vi "ProgramGlobalReg.vi"(7 "Global Reg":u32[](array[numeric])=[68228136, 235670073, 4294967264, 4294967295, 4294967295, 511] format="%x", 8 "error in (no error)":errorcluster, 9 "ChipID":u32=65535 format="%x", 10 "LayerID":u32=65535 format="%x", 11 "connection ID":refnum<k5>) -> (0 "error out":errorcluster, 1 "OK?":bool, 2 "GlobalReg programmed":u32[](array[numeric]) format="%08x", 3 "connection ID out":refnum<k5>, 4 "Program done":string[](array[string]))   [LabVIEW 2015, in "VIPM2.lvlib"]
doc: "Fa la comprovació en tots els casos (emmascarant els ChipIDs)."
uses:
  VIPM2.lvlib
panel:
  out "Ready to receive data":string
  # "Program Global Register"
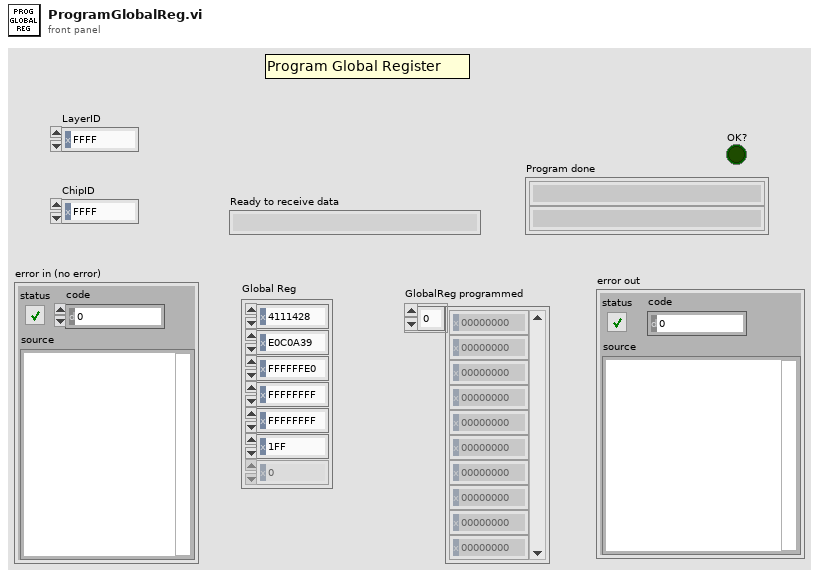
[diagram p1: front panel]
types:
  T1 = enum16{"Standard", "Buffered", "CRLF", "Immediate"}
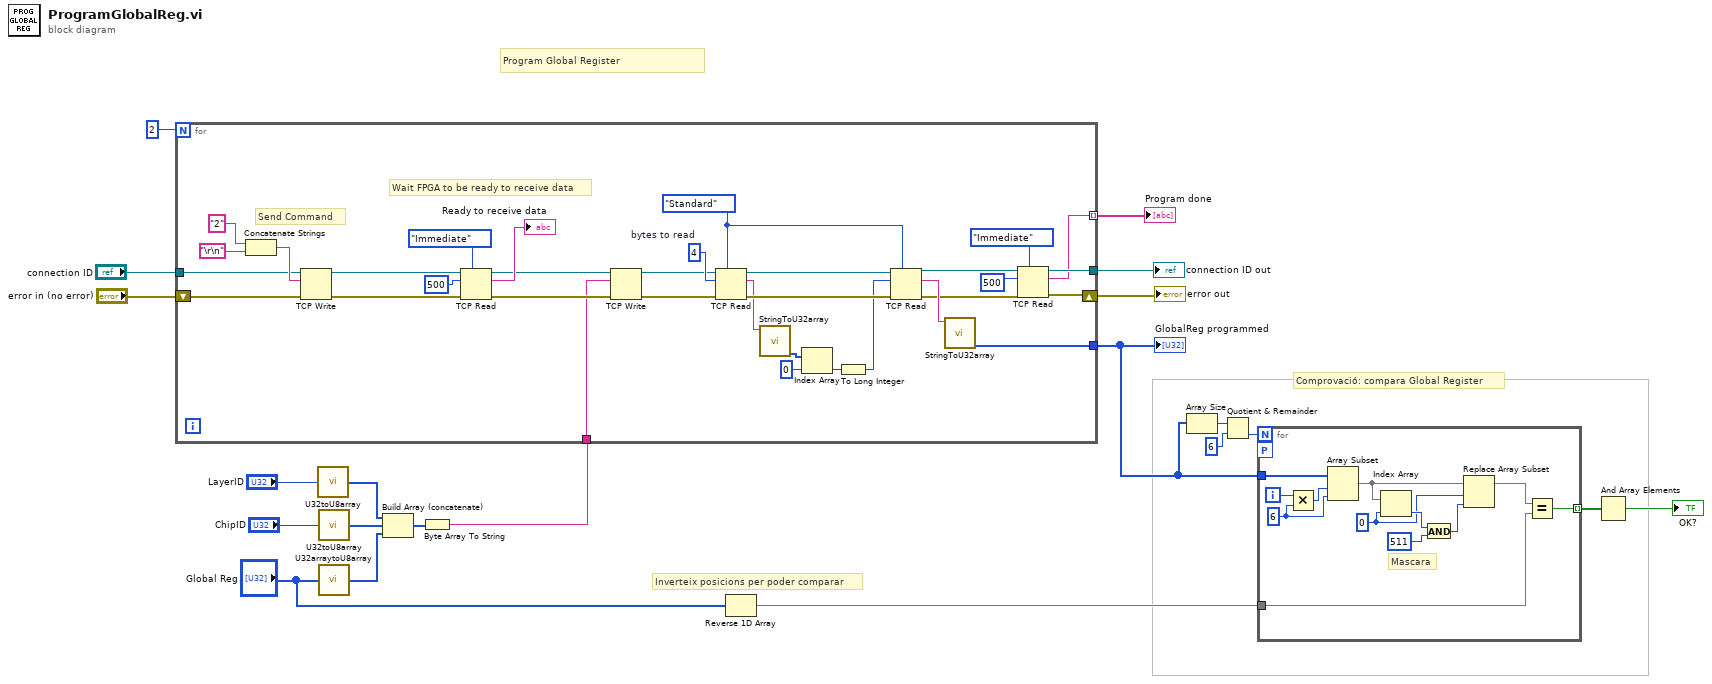
[diagram p0: block diagram]
diagram:
  # "Comprovació: compara Global Register"
  # "Inverteix posicions per poder comparar"
  # "Program Global Register"
  n1 = call "U32toU8array.vi"("x"="LayerID") -> ("ArrayU8"=w17:u8[])
  n2 = call "U32toU8array.vi"("x"="ChipID") -> ("ArrayU8"=w16:u8[])
  n3 = call "U32arraytoU8array.vi"("ArrayU32"="Global Reg") -> ("ArrayU8"=w15:u8[])
  n4 = Build Array (concatenate)(w17, w16, w15) -> (w18:u8[])
  n5 = Byte Array To String(unsigned byte array=w18) -> (string=w14:string)
  n6 = for {
    N: 2 -> [_]
    tunnel: "connection ID" -> [w51]
    tunnel: [w43] -> w20
    tunnel: [w42] -> w11 mode=indexing
    tunnel: w14 -> [w39]
    shift-right: [w25] -> w12
    shift-left: "error in (no error)" -> [w26]
    tunnel: [w24] -> w9
    w34 = 4  # bytes to read
    w35 = T1."Standard" ("mode (standard)")
    # "Wait FPGA to be ready to receive data"
    # "Send Command"
    n7 = Concatenate Strings("2" ("string"), "\r\n") -> (w52:string)
    n8 = TCP Write(connection ID=w51, data in=w52, error in (no error)=w26) -> (connection ID out=w47:refnum<k5>, error out=w46:errorcluster)  [unwired: 1 in, 1 out]
    n9 = TCP Read(connection ID=w47, bytes to read=500, error in (no error)=w46, 7:T1."Immediate" ("mode (standard)")) -> (connection ID out=w41:refnum<k5>, data out=→"Ready to receive data":string, error out=w40:errorcluster)  [unwired: 1 in]
    n10 = TCP Write(connection ID=w41, data in=w39, error in (no error)=w40) -> (connection ID out=w32:refnum<k5>, error out=w33:errorcluster)  [unwired: 1 in, 1 out]
    n11 = TCP Read(connection ID=w32, bytes to read=w34, error in (no error)=w33, 7:w35) -> (connection ID out=w38:refnum<k5>, data out=w31:string, error out=w37:errorcluster)  [unwired: 1 in]
    n12 = call "StringToU32array.vi"("String"=w31) -> ("U32array"=w30:u32[])  [unwired: 2 out]
    n13 = Index Array(array=w30, index=0) -> (element=w23:u32)
    n14 = To Long Integer(number=w23) -> (32bit integer=w22:i32)
    n15 = TCP Read(connection ID=w38, bytes to read=w22, error in (no error)=w37, 7:w35) -> (connection ID out=w28:refnum<k5>, data out=w29:string, error out=w27:errorcluster)  [unwired: 1 in]
    n16 = call "StringToU32array.vi"("String"=w29) -> ("U32array"=w24:u32[])  [unwired: 2 out]
    n17 = TCP Read(connection ID=w28, bytes to read=500, error in (no error)=w27, 7:T1."Immediate" ("mode (standard)")) -> (connection ID out=w43:refnum<k5>, data out=w42:string, error out=w25:errorcluster)  [unwired: 1 in]
  }
  "connection ID out" <- w20
  "error out" <- w12
  "Program done" <- w11
  "GlobalReg programmed" <- w9
  n18 = Reverse 1D Array(array="Global Reg") -> (reversed array=w6:u32[])
  n19 = Array Size(array=w9) -> (size(s)=w4:i32)
  n20 = Quotient & Remainder(x=w4, y=6) -> (floor(x/y)=w3:i32)  [unwired: 1 out]
  n21 = for {
    N: w3 -> [_]
    tunnel: w9 -> [w66]
    tunnel: w6 -> [w63]
    tunnel: [w62] -> w1 mode=indexing
    workers-P: _ -> [_]
    i -> [w56]
    w58 = 0 ("index")
    w55 = 6 ("length")
    # "Mascara"
    n22 = Multiply(x=w56, y=w55) -> (x*y=w57:i32)
    n23 = Array Subset "Array Subset"(array=w66, index=w57, length=w55) -> (w65:u32[])
    n24 = Index Array(array=w65, index=w58) -> (element=w61:u32)
    n25 = And(x=w61, y=u32 511) -> (x .and. y?=w59:u32)
    n26 = Replace Array Subset "Replace Array Subset"(array=w65, new element=w59, index=w58) -> (w64:u32[])
    n27 = Equal?(x=w64, y=w63) -> (x = y?=w62:bool)
  }
  n28 = And Array Elements(Boolean array=w1) -> (logical AND=→"OK?":bool)
